vi "SngJntArmSim_Pack_Model_Params.vi"(5 "DCMOTOR_TYPES":T2, 6 "Estimate MOI":bool, 7 "Num Motors":i32, 8 "MOI kgm2":dbl, 9 "Gearing":dbl, 10 "massKg":dbl, 11 "ArmLength_M":dbl) -> (3 "SngJntArmSim_Model _Params":T1 {"MOI kgm2" format="%#_13g"; "Gearing" format="%#_13g"; "massKg" format="%#_13g"; "ArmLength_M" format="%#_13g"})   [LabVIEW 2019, in "Trajectory_Library.lvlib"]
uses:
  Trajectory_Library.lvlib
  Enum/DCMOTOR_TYPES_ENUM.ctl
  TypeDef/SINGLE_JOINT_ARM_SIM_MODEL_PARAMS.ctl
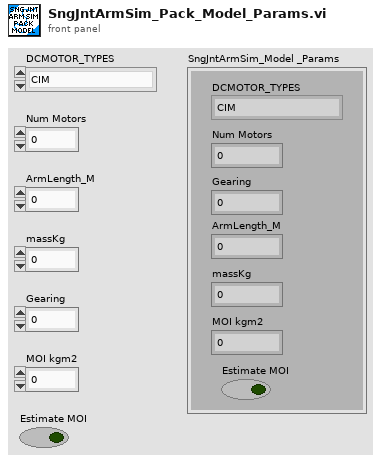
[diagram p1: front panel]
types:
  T1 = typedef "Trajectory_Library.lvlib/SINGLE_JOINT_ARM_SIM_MODEL_PARAMS.ctl" = cluster{"DCMOTOR_TYPES":T2, "Num Motors":i32, "ArmLength_M":dbl, "massKg":dbl, "Gearing":dbl, "MOI kgm2":dbl, "Estimate MOI":bool}
  T2 = typedef "Trajectory_Library.lvlib/DCMOTOR_TYPES_ENUM.ctl" = enum16{"CIM", "AndyMark 9015", "Andy Mark RS 775 125", "Bag", "BaneBots RS 550", "BaneBots RS 775", "Falcon 500", "Mini CIM", "NEO", "NEO 550", "Romi BuiltIn", "Vex 775 Pro", "Snow Blower AM 2235A", "Bosch Seat AM 3493"}
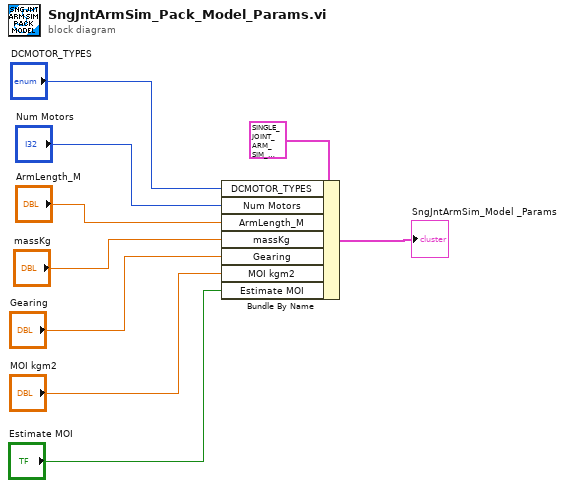
[diagram p0: block diagram]
diagram:
  n1 = Bundle By Name(cluster=T1 {"DCMOTOR_TYPES"=enum."NEO", "Num Motors"=1, "ArmLength_M"=0.75, "massKg"=26.0, "Gearing"=128.0, "MOI kgm2"=26.0, "Estimate MOI"=TRUE} ("SngJntArmSim_Model _Params"), "DCMOTOR_TYPES"="DCMOTOR_TYPES", "Num Motors"="Num Motors", "ArmLength_M"="ArmLength_M", "massKg"="massKg", "Gearing"="Gearing", "MOI kgm2"="MOI kgm2", "Estimate MOI"="Estimate MOI") -> (→"SngJntArmSim_Model _Params":T1)
